vi "update obstacle array.vi"(9 "Game Parameters":T3={"Upper Limit (m)"=100.0, "Lower Limit (m)"=0.0, "Obstacle time"=20.0, "Obstacle length"=10.0, "fuel decrement"=0.5, "Fuel time"=100.0, "fuel amount"=50.0, "Fuel range"=10, "Death range"=5, "Terrain slope"=35.0, "Speed (km/hr)"=150.0, "Time step (ms)"=30, "Gravity"=-9.81, "Date"="11/03/2016", "High scores path"=path "C:/Users/lz2/Code/LabVIEW/Helicopter/hi scores.txt", "Difficulty"=enum."Normal", "Headstart"=30}, 10 "loop counter":i32, 11 "Arrays and Heights":T1={"Score Array"=[], "Lowest high score"=0.0, "Score"=0.0, "Ceiling"=0.0, "Floor"=0.0, "Ceiling Array"=[], "Floor array"=[], "Helicopter height"=0.0, "Helicopter array"=[], "Fuel"=300.0, "Fuel array"=[], "fuel counter"=0, "obstacle counter"=0, "Obstacle array"=[], "helicopter v_0"=0.0, "helicopter a_0"=0.0, "Obstacle height"=300.0}) -> (3 "Arrays and heights":T1={"Score Array"=[], "Lowest high score"=0.0, "Score"=0.0, "Ceiling"=0.0, "Floor"=0.0, "Ceiling Array"=[], "Floor array"=[], "Helicopter height"=0.0, "Helicopter array"=[], "Fuel"=300.0, "Fuel array"=[], "fuel counter"=0, "obstacle counter"=0, "Obstacle array"=[], "helicopter v_0"=0.0, "helicopter a_0"=0.0, "Obstacle height"=300.0})   [LabVIEW 2017]
uses:
  controls/game parameters.ctl
  controls/arrays and heights.ctl
  controls/scores.ctl
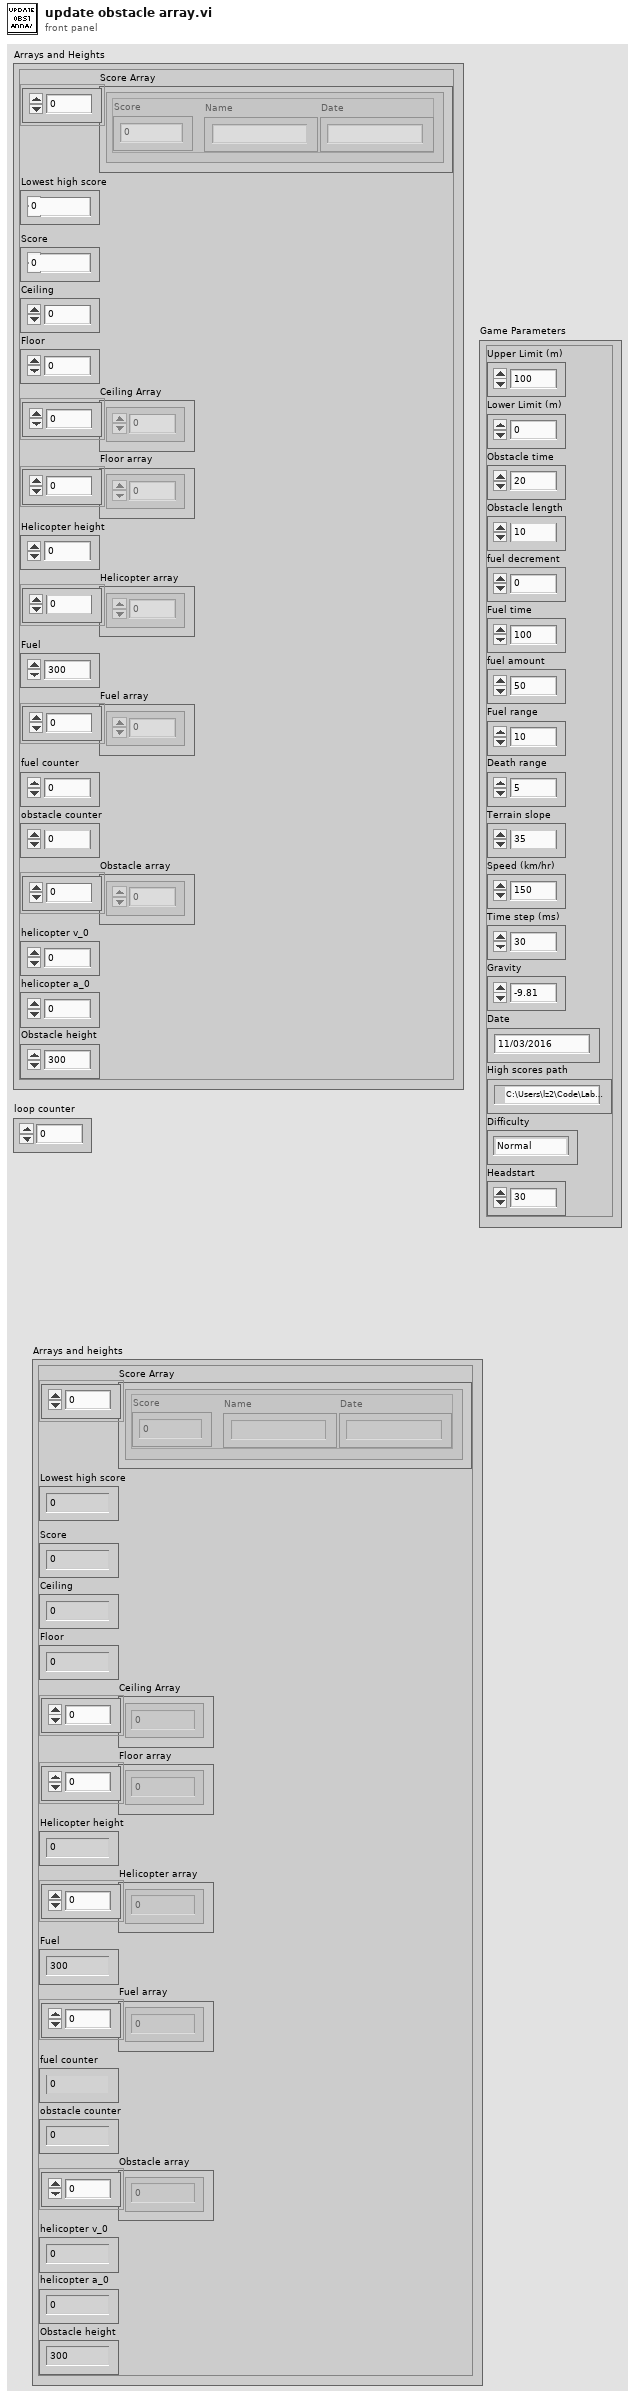
[diagram p1: front panel]
types:
  T1 = typedef "arrays and heights.ctl" = cluster{"Score Array":T2[], "Lowest high score":dbl, "Score":dbl, "Ceiling":dbl, "Floor":dbl, "Ceiling Array":dbl[], "Floor array":dbl[], "Helicopter height":dbl, "Helicopter array":dbl[], "Fuel":dbl, "Fuel array":dbl[], "fuel counter":i32, "obstacle counter":i32, "Obstacle array":dbl[], "helicopter v_0":dbl, "helicopter a_0":dbl, "Obstacle height":dbl}
  T2 = typedef "scores.ctl" = cluster{"Score":dbl, "Name":string, "Date":string}
  T3 = typedef "game parameters.ctl" = cluster{"Upper Limit (m)":dbl, "Lower Limit (m)":dbl, "Obstacle time":dbl, "Obstacle length":dbl, "fuel decrement":dbl, "Fuel time":dbl, "fuel amount":dbl, "Fuel range":i32, "Death range":i32, "Terrain slope":dbl, "Speed (km/hr)":dbl, "Time step (ms)":u32, "Gravity":dbl, "Date":string, "High scores path":path, "Difficulty":enum16{"Easy", "Normal", "Hard"}, "Headstart":u32}
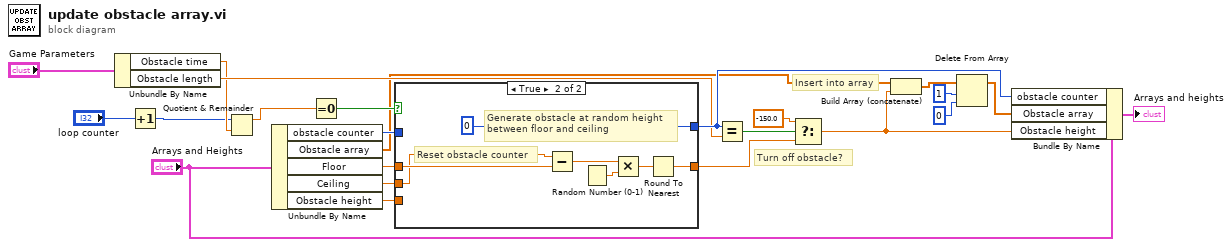
[diagram p0: block diagram]
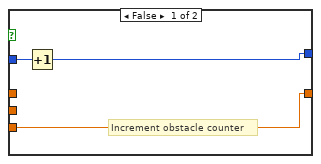
[diagram p2: hidden frame]
diagram:
  # "Insert into array"
  # "Turn off obstacle?"
  n1 = Unbundle By Name("Game Parameters") -> ("Obstacle time"=w16:dbl, "Obstacle length"=w18:dbl)
  n2 = Increment(x="loop counter") -> (x+1=w1:i32)
  n3 = Quotient & Remainder(x=w1, y=w16) -> (x-y*floor(x/y)=w15:dbl)  [unwired: 1 out]
  n4 = Unbundle By Name("Arrays and Heights") -> ("obstacle counter"=w13:i32, "Obstacle array"=w10:dbl[], "Floor"=w8:dbl, "Ceiling"=w7:dbl, "Obstacle height"=w2:dbl)
  n5 = Equal To 0?(x=w15) -> (x = 0?=w14:bool)
  n6 = case shown="True" w14 {
    tunnel: [w24 w31] -> w4
    tunnel: w13 -> [w26 _]
    tunnel: [w25 0] -> w19
    tunnel: w7 -> [_ w29]
    tunnel: w8 -> [_ w30]
    tunnel: w2 -> [w24 _]
    frame False {
      # "Increment obstacle counter"
      n7 = Increment(x=w26) -> (x+1=w25:i32)
    }
    frame True {
      # "Reset obstacle counter"
      # "Generate obstacle at random height\nbetween floor and ceiling"
      n8 = Subtract(x=w29, y=w30) -> (x-y=w28:dbl)
      n9 = Random Number (0-1)() -> (number: 0 to 1=w33:dbl)
      n10 = Multiply(x=w28, y=w33) -> (x*y=w27:dbl)
      n11 = Round To Nearest(number=w27) -> (nearest integer value=w31:dbl)
    }
  }
  n12 = Equal?(x=w19, y=w18) -> (x = y?=w6:bool)
  n13 = Select(t=-150.0 ("y"), s=w6, f=w4) -> (s? t:f=w3:dbl)
  n14 = Build Array (concatenate)(w10, w3) -> (w23:dbl[])
  n15 = Delete From Array(array=w23, length=1, index=0) -> (array with subset deleted=w11:dbl[])  [unwired: 1 out]
  n16 = Bundle By Name(cluster="Arrays and Heights", "obstacle counter"=w19, "Obstacle array"=w11, "Obstacle height"=w3) -> (→"Arrays and heights":T1)
